vi "1 - Queue driven state machine.vi"() -> ()   [LabVIEW 2015]
panel:
  out "On Off Indicator":bool
  out "Dirrection indicator":enum16{"Forward", "Reverse"}(ring)
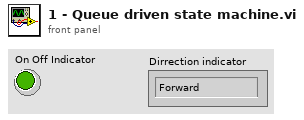
[diagram p1: front panel]
types:
  T1 = cluster{"Command":string, "Data":enum16{"Forward", "Reverse"}}
  T2 = cluster{"Speed":dbl, "Direction":enum16{"Forward", "Reverse"}, "On?":bool}
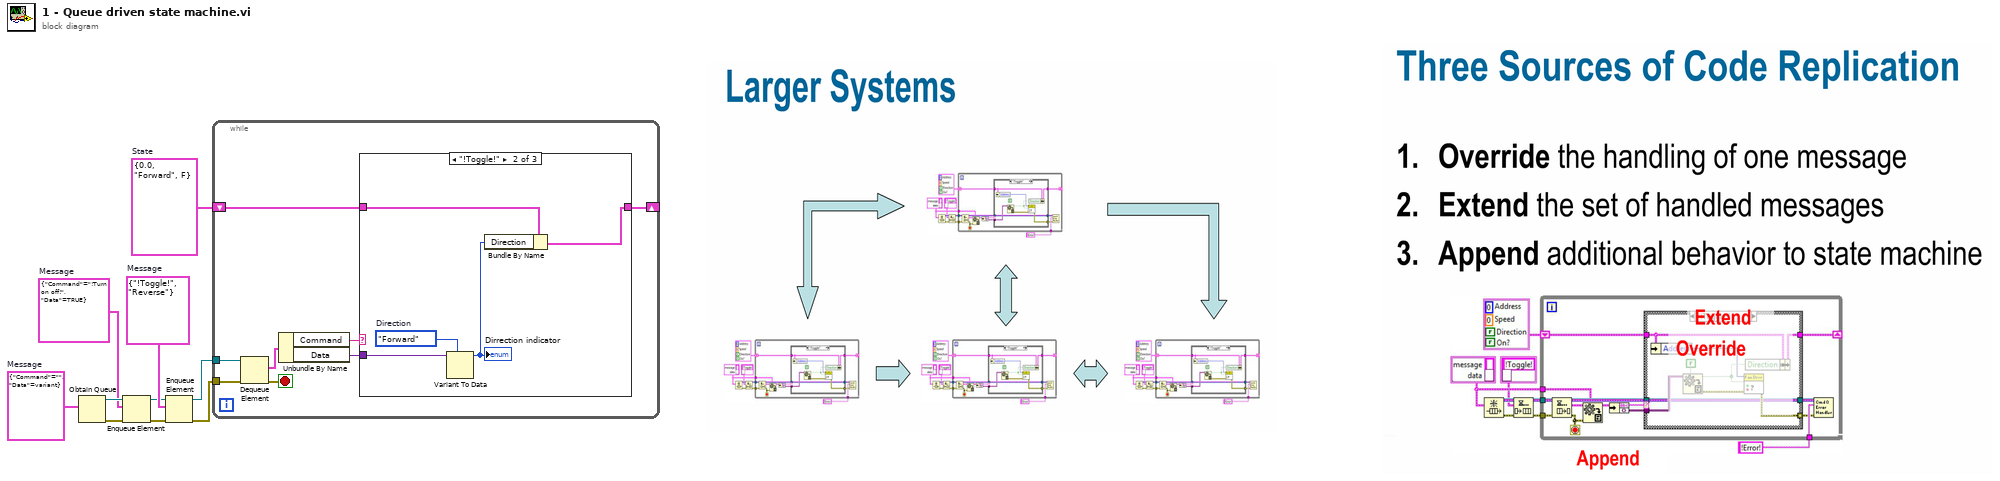
[diagram p0: block diagram]
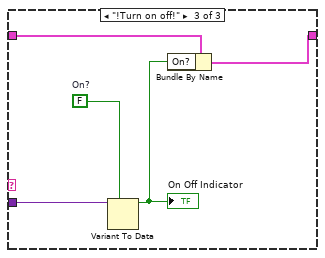
[diagram p3: hidden frame]
diagram:
  w1 = cluster{"Command":string, "Data":bool} {"Command"="!Turn on off!", "Data"=TRUE}  # Message
  w9 = T1 {"Command"="!Toggle!", "Data"=enum."Reverse"}  # Message
  w10 = cluster{"Command":string, "Data":variant} {"Command"="", "Data"=variant}  # Message
  w6 = T2 {"Speed"=0.0, "Direction"=enum."Forward", "On?"=FALSE}  # State
  n1 = Obtain Queue(element data type=w10) -> (queue out=w3:refnum<queue>, error out=w5:errorcluster)  [unwired: 4 in, 1 out]
  n2 = Enqueue Element(queue=w3, element=w1, error in (no error)=w5) -> (queue out=w2:refnum<queue>, error out=w4:errorcluster)  [unwired: 1 in, 1 out]
  n3 = Enqueue Element(queue=w2, element=w9, error in (no error)=w4) -> (queue out=w7:refnum<queue>, error out=w8:errorcluster)  [unwired: 1 in, 1 out]
  n4 = while {
    tunnel: w8 -> [w18]
    tunnel: w7 -> [w17]
    shift-right: [w11] -> _
    shift-left: w6 -> [w12]
    stop <- w15 stop-if-true
    n5 = Dequeue Element(queue=w17, error in (no error)=w18) -> (element=w16:cluster{"Command":string, "Data":variant}, error out=w15:errorcluster)  [unwired: 1 in, 2 out]
    n6 = Unbundle By Name(w16) -> ("Command"=w14:string, "Data"=w13:variant)
    n7 = case shown="\"!Toggle!\"" w14 {
      tunnel: w13 -> [_ w24 w29]
      tunnel: w12 -> [w19 w22 w28]
      tunnel: [w19 w20 w27] -> w11
      frame "\u0000", Default {
      }
      frame "!Toggle!" {
        w23 = enum16{"Forward", "Reverse"}."Forward"  # Direction
        n8 = Variant To Data(type=w23, Variant=w24) -> (data=w21:enum16{"Forward", "Reverse"})  [unwired: 1 in, 1 out]
        "Dirrection indicator" <- w21
        n9 = Bundle By Name(cluster=w22, "Direction"=w21) -> (w20:T2)
      }
      frame "!Turn on off!" {
        w26 = FALSE  # On?
        n10 = Variant To Data(type=w26, Variant=w29) -> (data=w25:bool)  [unwired: 1 in, 1 out]
        "On Off Indicator" <- w25
        n11 = Bundle By Name(cluster=w28, "On?"=w25) -> (w27:T2)
      }
    }
  }
